vi "Flow_Guide-plot.vi"(6 "Time In":i32, 8 "Temperature Sync":i32, 9 "Temp Band % (e.g. 1%=1.01)":dbl=1.04, 10 "Mean(Off)/Interval(On)":bool, 11 "Guide":bool) -> (2 "Graph 2":dbl, 3 "Graph 1":dbl, 4 "Time out":i32)   [LabVIEW 2014]
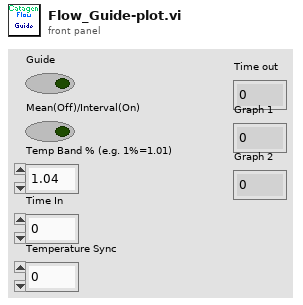
[diagram p1: front panel]
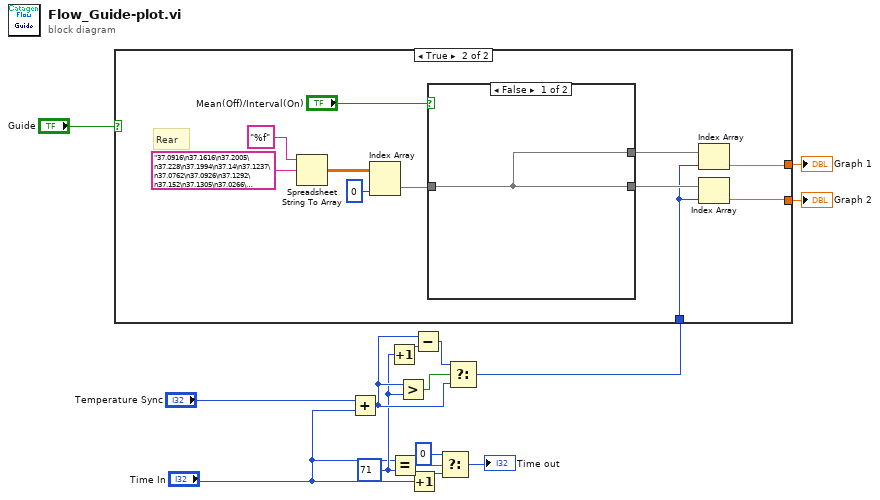
[diagram p0: block diagram]
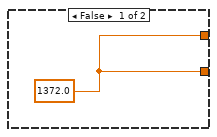
[diagram p2: hidden frame]
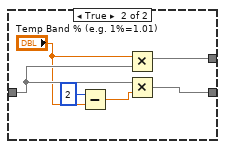
[diagram p3: hidden frame]
diagram:
  w6 = 71 ("y")
  n1 = Add(x="Temperature Sync", y="Time In") -> (x+y=w8:i32)
  n2 = Increment(x=w6) -> (x+1=w7:i32)
  n3 = Equal?(x="Time In", y=w6) -> (x = y?=w13:bool)
  n4 = Greater?(x=w8, y=w6) -> (0:w10:bool)
  n5 = Increment(x="Time In") -> (x+1=w11:i32)
  n6 = Subtract(x=w8, y=w7) -> (x-y=w9:i32)
  n7 = Select(t=0, s=w13, f=w11) -> (s? t:f=→"Time out":i32)
  n8 = Select(t=w9, s=w10, f=w8) -> (s? t:f=w5:i32)
  n9 = case shown="True" "Guide" {
    tunnel: w5 -> [_ w17]
    tunnel: [w16 w18] -> w2
    tunnel: [w16 w19] -> w1
    frame False {
      w16 = 1372.0
    }
    frame True {
      # "Rear"
      n10 = Spreadsheet String To Array(format string="%f", spreadsheet string="37.0916\n37.1616\n37.2005\n37.228\n37.1994\n37.14\n37.1237\n37.0762\n37.0926\n37.1292\n37.152\n37.1305\n37.0266\n36.8432\n36.7674\n36.6781\n36.6541\n36.7295\n36.8392\n36.8699\n36.7399\n32.4831\n13.3192\n3.7366\n2.2297\n2.0056\n1.9387\n1.7048\n1.5939\n9.8865\n28.4264\n35.117\n35.7585\n35.9395\n36.1823\n36.3668\n36.5273\n36.6775\n36.771\n36.8306\n36.8585\n36.9024\n36.9508\n37.0343\n37.108\n37.144\n37.0359\n36.9294\n36.8464\n36.7377\n36.7104\n36.7562\n36.8583\n36.9636\n36.9884\n37.0251\n36.8451\n36.3171\n25.9636\n7.657\n2.4983\n2.1837\n1.947\n1.7619\n1.6701\n10.7561\n29.4948\n36.0944\n36.8921\n37.1834\n36.9375\n36.9317") -> (array=w25:dbl[][])  [unwired: 2 in]
      n11 = Index Array(array=w25, index (col)=0 ("disabled index (col)")) -> (element=w23:dbl[])  [unwired: 1 in]
      n12 = case shown="False" "Mean(Off)/Interval(On)" {
        tunnel: w23 -> [w28 w31]
        tunnel: [w28 w32] -> w21
        tunnel: [w28 w33] -> w20
        frame False {
        }
        frame True {
          n13 = Subtract(x=2, y="Temp Band % (e.g. 1%=1.01)") -> (x-y=w29:dbl)
          n14 = Multiply(x="Temp Band % (e.g. 1%=1.01)", y=w31) -> (x*y=w33:dbl[])
          n15 = Multiply(x=w31, y=w29) -> (x*y=w32:dbl[])
        }
      }
      n16 = Index Array(array=w20, index=w17) -> (element=w18:dbl)
      n17 = Index Array(array=w21, index=w17) -> (element=w19:dbl)
    }
  }
  "Graph 1" <- w2
  "Graph 2" <- w1
